vi "LoadJoystickImages.vi"(11 "UiDefinition 2":T1) -> ()   [LabVIEW 2020]
uses:
  UIReferences.ctl
  C:/Users/User/Desktop/Automation/NextVersion2/LabviewDXFViewer/bin/Release/LabviewDXFViewer.exe
  LabviewDXFViewer/bin/Release/LabviewDXFViewer.exe
panel:
  in  "image":i32(ring)=13 items=["Left", "LeftBig", "LeftSmall", "Right", "RightBig", "RightSmall", "Up", "UpBig", "UpSmall", "Down", "DownBig", "DownSmall", "Zero", "Play", "Pause", "Load", "Lower", "Raise", "Home", "Home2"]
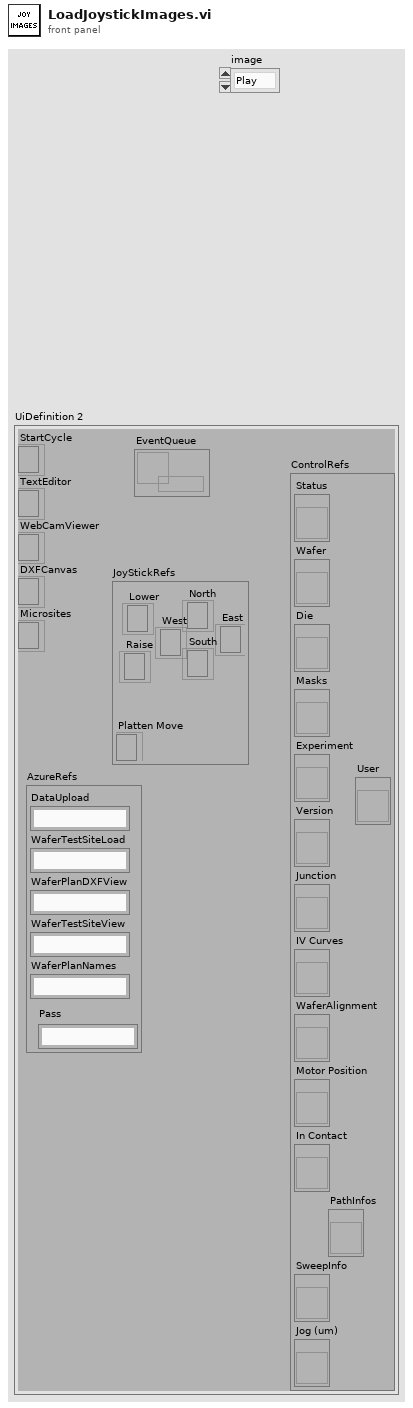
[diagram p1: front panel]
types:
  T1 = typedef "UIReferences.ctl" = cluster{"StartCycle":refnum<k24>, "TextEditor":refnum<k24>, "WebCamViewer":refnum<k24>, "DXFCanvas":refnum<k24>, "Microsites":refnum<k24>, "JoyStickRefs":cluster{"North":refnum<k24>, "Lower":refnum<k24>, "Raise":refnum<k24>, "Platten Move":refnum<k24>, "West":refnum<k24>, "East":refnum<k24>, "South":refnum<k24>}, "AzureRefs":cluster{"DataUpload":string, "WaferTestSiteLoad":string, "WaferPlanDXFView":string, "WaferTestSiteView":string, "WaferPlanNames":string, "Pass":string}, "ControlRefs":cluster{"Status":refnum<vi>, "Wafer":refnum<vi>, "Die":refnum<vi>, "Masks":refnum<vi>, "Experiment":refnum<vi>, "Version":refnum<vi>, "Junction":refnum<vi>, "IV Curves":refnum<vi>, "WaferAlignment":refnum<vi>, "Motor Position":refnum<vi>, "In Contact":refnum<vi>, "SweepInfo":refnum<vi>, "Jog (um)":refnum<vi>, "PathInfos":refnum<vi>, "User":refnum<vi>}, "EventQueue":refnum<queue>}
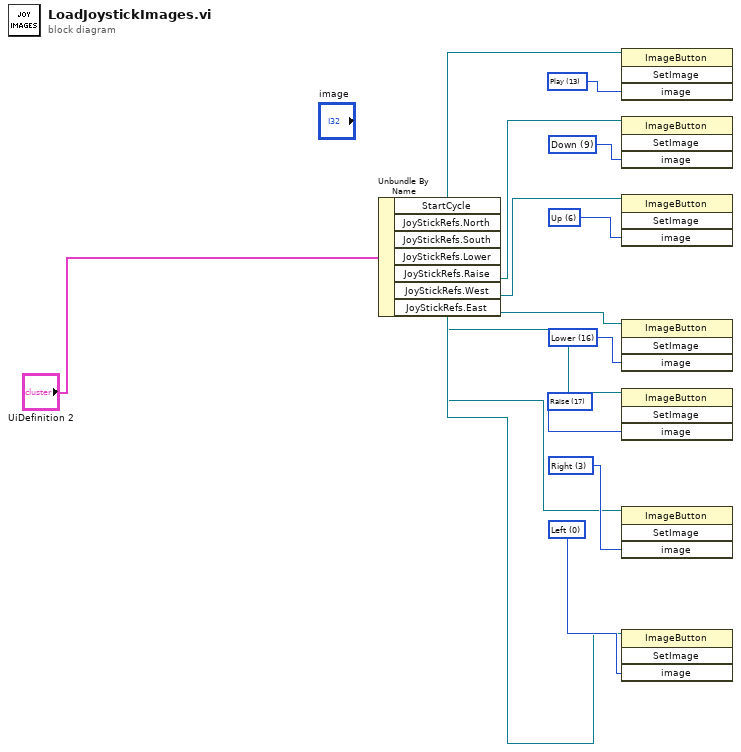
[diagram p0: block diagram]
diagram:
  w15 = 13 items=["Left", "LeftBig", "LeftSmall", "Right", "RightBig", "RightSmall", "Up", "UpBig", "UpSmall", "Down", "DownBig", "DownSmall", "Zero", "Play", "Pause", "Load", "Lower", "Raise", "Home", "Home2"] ("image")
  w14 = 0 items=["Left", "LeftBig", "LeftSmall", "Right", "RightBig", "RightSmall", "Up", "UpBig", "UpSmall", "Down", "DownBig", "DownSmall", "Zero", "Play", "Pause", "Load", "Lower", "Raise", "Home", "Home2"] ("image")
  w13 = 3 items=["Left", "LeftBig", "LeftSmall", "Right", "RightBig", "RightSmall", "Up", "UpBig", "UpSmall", "Down", "DownBig", "DownSmall", "Zero", "Play", "Pause", "Load", "Lower", "Raise", "Home", "Home2"] ("image")
  w12 = 17 items=["Left", "LeftBig", "LeftSmall", "Right", "RightBig", "RightSmall", "Up", "UpBig", "UpSmall", "Down", "DownBig", "DownSmall", "Zero", "Play", "Pause", "Load", "Lower", "Raise", "Home", "Home2"] ("image")
  w11 = 16 items=["Left", "LeftBig", "LeftSmall", "Right", "RightBig", "RightSmall", "Up", "UpBig", "UpSmall", "Down", "DownBig", "DownSmall", "Zero", "Play", "Pause", "Load", "Lower", "Raise", "Home", "Home2"] ("image")
  w10 = 6 items=["Left", "LeftBig", "LeftSmall", "Right", "RightBig", "RightSmall", "Up", "UpBig", "UpSmall", "Down", "DownBig", "DownSmall", "Zero", "Play", "Pause", "Load", "Lower", "Raise", "Home", "Home2"] ("image")
  w4 = 9 items=["Left", "LeftBig", "LeftSmall", "Right", "RightBig", "RightSmall", "Up", "UpBig", "UpSmall", "Down", "DownBig", "DownSmall", "Zero", "Play", "Pause", "Load", "Lower", "Raise", "Home", "Home2"] ("image")
  n1 = Unbundle By Name("UiDefinition 2") -> ("StartCycle"=w1:refnum<k24>, "JoyStickRefs.North"=w3:refnum<k24>, "JoyStickRefs.South"=w5:refnum<k24>, "JoyStickRefs.Lower"=w6:refnum<k24>, "JoyStickRefs.Raise"=w7:refnum<k24>, "JoyStickRefs.West"=w8:refnum<k24>, "JoyStickRefs.East"=w9:refnum<k24>)
  n2 = invoke class="ImageButton" method="SetImage"(reference=w1, "image"=w15) -> ()  [unwired: 2 in, 4 out]
  n3 = invoke class="ImageButton" method="SetImage"(reference=w3, "image"=w4) -> ()  [unwired: 2 in, 4 out]
  n4 = invoke class="ImageButton" method="SetImage"(reference=w5, "image"=w10) -> ()  [unwired: 2 in, 4 out]
  n5 = invoke class="ImageButton" method="SetImage"(reference=w6, "image"=w11) -> ()  [unwired: 2 in, 4 out]
  n6 = invoke class="ImageButton" method="SetImage"(reference=w7, "image"=w12) -> ()  [unwired: 2 in, 4 out]
  n7 = invoke class="ImageButton" method="SetImage"(reference=w8, "image"=w13) -> ()  [unwired: 2 in, 4 out]
  n8 = invoke class="ImageButton" method="SetImage"(reference=w9, "image"=w14) -> ()  [unwired: 2 in, 4 out]
